vi "Init.vi"(8 "error in (no error)":errorcluster, 11 "Path":path) -> (0 "error out":errorcluster, 3 "Config-YAML out":refnum<class "Config-YAML.lvclass">)   [LabVIEW 2020, in "CDM-Config.lvlib" / "Config-YAML.lvclass"]
uses:
  Config-YAML.lvclass
  Config-YAML.lvclass/Config-YAML.ctl
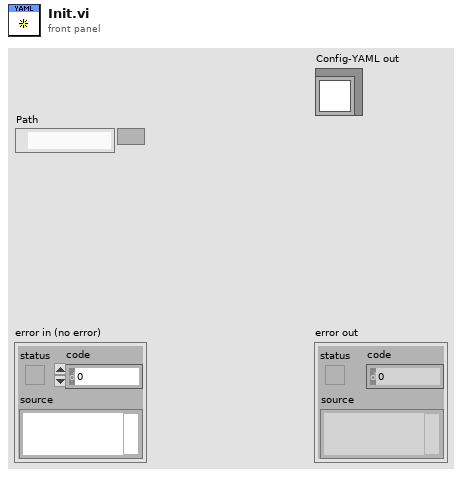
[diagram p1: front panel]
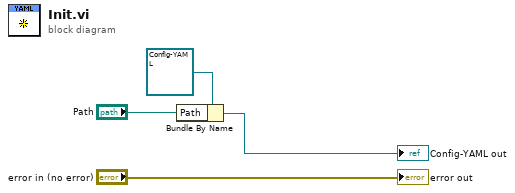
[diagram p0: block diagram]
diagram:
  n1 = Bundle By Name(cluster=refnum<class "Config-YAML.lvclass"> refnum ("Config-YAML in"), "Path"="Path") -> (→"Config-YAML out":refnum<class "Config-YAML.lvclass">)
  "error out" <- "error in (no error)"
